vi "Sandbox_RtVar.vi"() -> ()   [LabVIEW 2019, in "RT_Shared_Variables.lvlib"]
uses:
  RT_Shared_Variables.lvlib
  f094185d-fbc1-4b7f-a2b5-6bfc8c4f0055.vi
  <vilib>/Utility/Variable/NI_VariableUtilities.lvlib
panel:
  out "Numeric":i32
  out "error out":errorcluster
  out "read per mks":dbl format="%#_6p"
  out "dt":u32
  out "index":i32
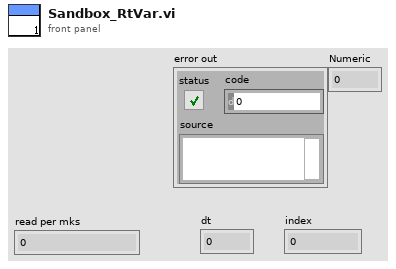
[diagram p1: front panel]
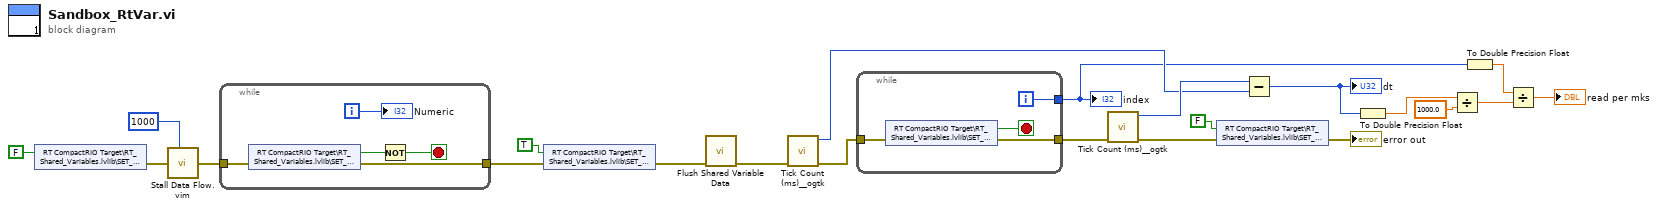
[diagram p0: block diagram]
diagram:
  n1 = shared-variable "RT CompactRIO Target\\RT_Shared_Variables.lvlib\\SET_CONFIG"(FALSE ("SET_CONFIG")) -> (error out=w21:errorcluster)  [unwired: 1 in]
  n2 = call "Stall Data Flow.vim"("value in"=w21, "milliseconds to wait"=u32 1000) -> ("value out"=w2:errorcluster)  [unwired: 1 out]
  n3 = while {
    tunnel: w2 -> [w27]
    tunnel: [w24] -> w19
    i -> [w23]
    stop <- w25 stop-if-true
    n4 = shared-variable "RT CompactRIO Target\\RT_Shared_Variables.lvlib\\SET_CONFIG"(error in=w27) -> (w26:bool, error out=w24:errorcluster)
    n5 = Not(x=w26) -> (.not. x?=w25:bool)
    "Numeric" <- w23
  }
  n6 = shared-variable "RT CompactRIO Target\\RT_Shared_Variables.lvlib\\SET_CONFIG"(TRUE ("SET_CONFIG"), error in=w19) -> (error out=w7:errorcluster)
  n7 = call <vilib>:"Flush Shared Variable Data.vi"("error in (no error)"=w7) -> ("error out"=w6:errorcluster)  [unwired: 10 in]
  n8 = call <userlib>:"Tick Count (ms)__ogtk.vi"("error in (no error)"=w6) -> ("error out"=w18:errorcluster, "millisecond timer value"=w15:u32)  [unwired: 9 in]
  n9 = while {
    tunnel: w18 -> [w30]
    tunnel: [w29] -> w13
    tunnel: [w28] -> w17
    i -> [w29]
    stop <- w31 stop-if-true
    n10 = shared-variable "RT CompactRIO Target\\RT_Shared_Variables.lvlib\\SET_CONFIG"(error in=w30) -> (w31:bool, error out=w28:errorcluster)
  }
  "index" <- w13
  n11 = call <userlib>:"Tick Count (ms)__ogtk.vi"("error in (no error)"=w17) -> ("error out"=w4:errorcluster, "millisecond timer value"=w16:u32)  [unwired: 9 in]
  n12 = shared-variable "RT CompactRIO Target\\RT_Shared_Variables.lvlib\\SET_CONFIG"(FALSE ("SET_CONFIG"), error in=w4) -> (error out=→"error out":errorcluster)
  n13 = Subtract(x=w16, y=w15) -> (x-y=w14:u32)
  "dt" <- w14
  n14 = To Double Precision Float(number=w14) -> (double precision float=w10:dbl)
  n15 = Divide(x=w10, y=1000.0 ("value")) -> (x/y=w8:dbl)
  n16 = To Double Precision Float(number=w13) -> (double precision float=w11:dbl)
  n17 = Divide(x=w11, y=w8) -> (x/y=→"read per mks":dbl)
